vi "Time_Date_Data.vi"(8 "error in (no error)":errorcluster, 10 "SQL date time In":string, 11 "Serial Number":string) -> (0 "error out":errorcluster, 1 "WeekYearCode":string, 2 "UTC ISO 8601":string, 3 "time stamp":timestamp format="%<%H:%M:%S\n%d/%m/%Y>T", 4 "BTW WWYYSN":string, 5 "date time rec":T1, 6 "Sql datetime type 20":string, 7 "EMA time":string)   [LabVIEW 2013]
uses:
  <vilib>/Utility/miscctls.llb/LVDateTimeRec.ctl
  Main Support/Global 2.vi
panel:
  # "YYYYMMDDThhmmssZ"
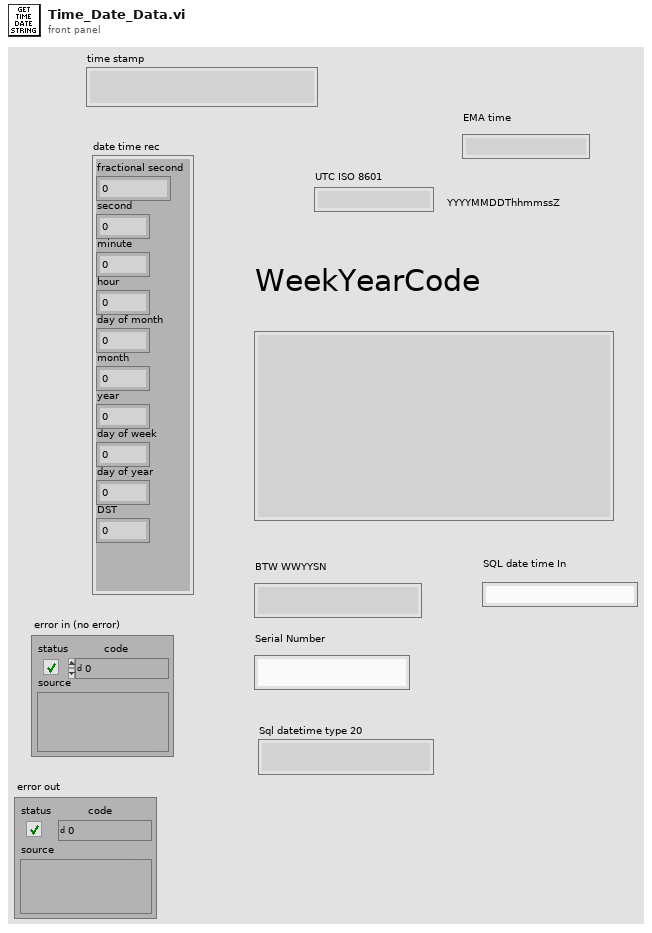
[diagram p1: front panel]
types:
  T1 = typedef "LVDateTimeRec.ctl" = cluster{"fractional second":dbl, "second":i32, "minute":i32, "hour":i32, "day of month":i32, "month":i32, "year":i32, "day of week":i32, "day of year":i32, "DST":i32}
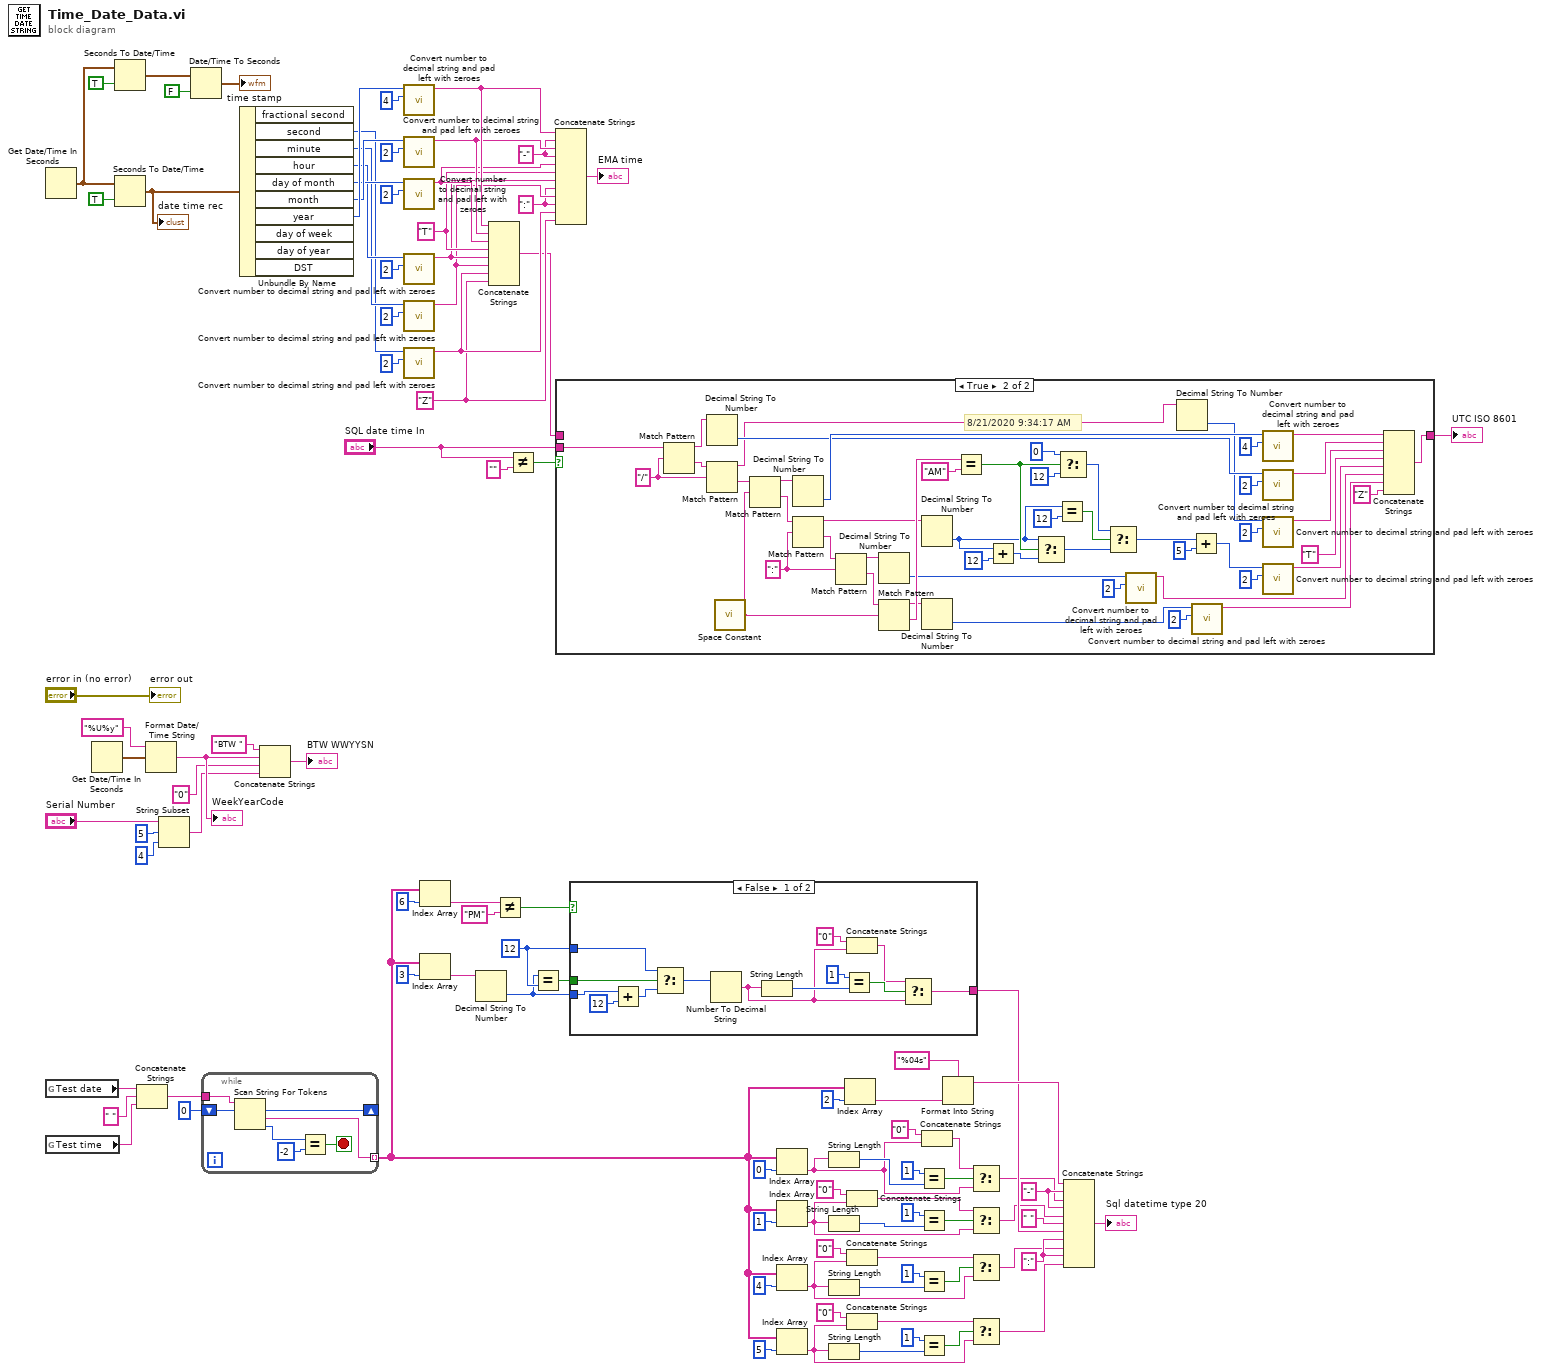
[diagram p0: block diagram]
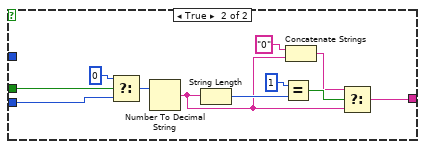
[diagram p3: hidden frame]
diagram:
  w9 = ":" ("string")
  w14 = "-" ("string")
  w50 = ":" ("string")
  w54 = "-" ("string")
  w56 = 12 ("y")
  w7 = "Z" ("string")
  w12 = "T" ("string")
  n1 = Get Date/Time In Seconds() -> (seconds since 1Jan1904=w96:timestamp)
  n2 = global read "Global 2.vi" "Test date"() -> (w20:string)
  n3 = global read "Global 2.vi" "Test time"() -> (w18:string)
  n4 = Get Date/Time In Seconds() -> (seconds since 1Jan1904=w94:timestamp)
  n5 = Seconds To Date/Time(time stamp (now)=w96, to UTC (F)=TRUE) -> (date time rec=w100:T1)
  n6 = Seconds To Date/Time(time stamp (now)=w96, to UTC (F)=TRUE) -> (date time rec=w95:T1)
  "date time rec" <- w95
  n7 = Concatenate Strings(w20, " " ("string"), w18) -> (w17:string)
  n8 = Format Date/Time String(time format string (%c)="%U%y", seconds (now)=w94) -> (date/time string=w91:string)  [unwired: 1 in]
  "WeekYearCode" <- w91
  n9 = String Subset(string="Serial Number", offset (0)=5, length (rest)=4 ("length (rest)")) -> (substring=w87:string)
  n10 = Date/Time To Seconds(1:FALSE ("to UTC (F)"), 2:w100) -> (0:→"time stamp":timestamp)
  n11 = while {
    tunnel: w17 -> [w109]
    shift-right: [w105] -> _
    shift-left: 0 -> [w106]
    tunnel: [w103] -> w61 mode=indexing
    stop <- w107 stop-if-true
    n12 = Scan String For Tokens(8:w106, 9:w109) -> (0:w104:i32, 1:w103:string, 2:w105:i32)  [unwired: 4 in, 1 out]
    n13 = Equal?(x=w104, y=-2) -> (x = y?=w107:bool)
  }
  n14 = Unbundle By Name(w95) -> ("second"=w74:i32, "minute"=w76:i32, "hour"=w78:i32, "day of month"=w80:i32, "month"=w82:i32, "year"=w84:i32)  [unwired: 4 out]
  n15 = Concatenate Strings("BTW " ("string"), w91, "0" ("string"), w87) -> (→"BTW WWYYSN":string)
  n16 = call "Convert number to decimal string and pad left with zeroes.vi"("Width"=u32 4, "number"=w84) -> ("result string"=w16:string)  [unwired: 9 in]
  n17 = call "Convert number to decimal string and pad left with zeroes.vi"("Width"=u32 2, "number"=w82) -> ("result string"=w15:string)  [unwired: 9 in]
  n18 = call "Convert number to decimal string and pad left with zeroes.vi"("Width"=u32 2, "number"=w80) -> ("result string"=w13:string)  [unwired: 9 in]
  n19 = call "Convert number to decimal string and pad left with zeroes.vi"("Width"=u32 2, "number"=w78) -> ("result string"=w11:string)  [unwired: 9 in]
  n20 = call "Convert number to decimal string and pad left with zeroes.vi"("Width"=i16 2 ("width (-)"), "number"=w76) -> ("result string"=w10:string)  [unwired: 9 in]
  n21 = call "Convert number to decimal string and pad left with zeroes.vi"("Width"=i16 2 ("width (-)"), "number"=w74) -> ("result string"=w8:string)  [unwired: 9 in]
  n22 = Index Array(array=w61, index=6) -> (element=w60:string)
  n23 = Index Array(array=w61, index=3) -> (element=w63:string)
  n24 = Decimal String To Number(string=w63) -> (number=w21:i32)  [unwired: 2 in, 1 out]
  n25 = Concatenate Strings(w16, w15, w13, w12, w11, w10, w8, w7) -> (w3:string)
  n26 = Not Equal?(x=w60, y="PM") -> (x != y?=w58:bool)
  n27 = Not Equal?(x="SQL date time In", y="") -> (x != y?=w4:bool)
  n28 = Equal?(x=w21, y=w56) -> (x = y?=w57:bool)
  n29 = Concatenate Strings(w16, w14, w15, w14, w13, w12, w11, w9, w10, w9, w8, w7) -> (→"EMA time":string)
  n30 = case shown="True" w4 {
    tunnel: w3 -> [w110 _]
    tunnel: [w110 w160] -> w2
    tunnel: "SQL date time In" -> [_ w158]
    frame False {
    }
    frame True {
      w152 = ":" ("regular expression")
      w156 = "/" ("regular expression")
      # "8/21/2020 9:34:17 AM"
      n31 = Match Pattern(string=w158, regular expression=w156) -> (before substring=w143:string, after substring=w157:string)  [unwired: 1 in, 2 out]
      n32 = Decimal String To Number(string=w143) -> (number=w145:i32)  [unwired: 2 in, 1 out]
      n33 = Match Pattern(string=w157, regular expression=w156) -> (before substring=w140:string, after substring=w155:string)  [unwired: 1 in, 2 out]
      n34 = call <vilib>:"Space Constant.vi"() -> ("String"=w150:string)
      n35 = Match Pattern(string=w155, regular expression=w150) -> (before substring=w147:string, after substring=w154:string)  [unwired: 1 in, 2 out]
      n36 = Decimal String To Number(string=w147) -> (number=w146:i32)  [unwired: 2 in, 1 out]
      n37 = Match Pattern(string=w154, regular expression=w152) -> (before substring=w138:string, after substring=w153:string)  [unwired: 1 in, 2 out]
      n38 = Match Pattern(string=w153, regular expression=w152) -> (before substring=w135:string, after substring=w151:string)  [unwired: 1 in, 2 out]
      n39 = Decimal String To Number(string=w135) -> (number=w137:i32)  [unwired: 2 in, 1 out]
      n40 = Match Pattern(string=w151, regular expression=w150) -> (before substring=w132:string, after substring=w149:string)  [unwired: 1 in, 2 out]
      n41 = Decimal String To Number(string=w138) -> (number=w116:i32)  [unwired: 2 in, 1 out]
      n42 = Decimal String To Number(string=w132) -> (number=w133:i32)  [unwired: 2 in, 1 out]
      n43 = Equal?(x=w149, y="AM") -> (x = y?=w117:bool)
      n44 = Add(x=w116, y=12) -> (x+y=w115:i32)
      n45 = Select(t=w116, s=w117, f=w115) -> (s? t:f=w114:i32)
      n46 = Equal?(x=w116, y=12) -> (x = y?=w122:bool)
      n47 = Select(t=u32 0 ("Width"), s=w117, f=12 ("y")) -> (s? t:f=w118:u32)
      n48 = Select(t=w118, s=w122, f=w114) -> (s? t:f=w111:u32)
      n49 = call "Convert number to decimal string and pad left with zeroes.vi"("Width"=u32 2, "number"=w137) -> ("result string"=w125:string)  [unwired: 9 in]
      n50 = Decimal String To Number(string=w140) -> (number=w141:i32)  [unwired: 2 in, 1 out]
      n51 = Add(x=w111, y=5) -> (x+y=w112:u32)
      n52 = call "Convert number to decimal string and pad left with zeroes.vi"("Width"=u32 2, "number"=w133) -> ("result string"=w124:string)  [unwired: 9 in]
      n53 = call "Convert number to decimal string and pad left with zeroes.vi"("Width"=u32 4, "number"=w146) -> ("result string"=w129:string)  [unwired: 9 in]
      n54 = call "Convert number to decimal string and pad left with zeroes.vi"("Width"=u32 2, "number"=w145) -> ("result string"=w128:string)  [unwired: 9 in]
      n55 = call "Convert number to decimal string and pad left with zeroes.vi"("Width"=u32 2, "number"=w141) -> ("result string"=w127:string)  [unwired: 9 in]
      n56 = call "Convert number to decimal string and pad left with zeroes.vi"("Width"=u32 2, "number"=w112) -> ("result string"=w126:string)  [unwired: 9 in]
      n57 = Concatenate Strings(w129, w128, w127, "T" ("string"), w126, w125, w124, "Z" ("string")) -> (w160:string)
    }
  }
  "UTC ISO 8601" <- w2
  n58 = case shown="False" w58 {
    tunnel: w57 -> [w173 w184]
    tunnel: w56 -> [w171 _]
    tunnel: [w162 w174] -> w52
    tunnel: w21 -> [w169 w182]
    frame False {
      n59 = Add(x=w169, y=12) -> (x+y=w172:i32)
      n60 = Select(t=w171, s=w173, f=w172) -> (s? t:f=w161:i32)
      n61 = Number To Decimal String(number=w161) -> (decimal integer string=w163:string)  [unwired: 1 in]
      n62 = String Length(string=w163) -> (length=w168:i32)
      n63 = Equal?(x=1, y=w168) -> (x = y?=w166:bool)
      n64 = Concatenate Strings("0" ("format string"), w163) -> (w164:string)
      n65 = Select(t=w164, s=w166, f=w163) -> (s? t:f=w162:string)
    }
    frame True {
      n66 = Select(t=i16 0 ("width (-)"), s=w184, f=w182) -> (s? t:f=w181:i32)
      n67 = Number To Decimal String(number=w181) -> (decimal integer string=w175:string)  [unwired: 1 in]
      n68 = String Length(string=w175) -> (length=w180:i32)
      n69 = Equal?(x=1, y=w180) -> (x = y?=w178:bool)
      n70 = Concatenate Strings("0" ("format string"), w175) -> (w176:string)
      n71 = Select(t=w176, s=w178, f=w175) -> (s? t:f=w174:string)
    }
  }
  n72 = Index Array(array=w61, index=0) -> (element=w44:string)
  n73 = Index Array(array=w61, index=1) -> (element=w37:string)
  n74 = Index Array(array=w61, index=4) -> (element=w30:string)
  n75 = Index Array(array=w61, index=5) -> (element=w23:string)
  n76 = String Length(string=w44) -> (length=w49:i32)
  n77 = String Length(string=w37) -> (length=w38:i32)
  n78 = String Length(string=w30) -> (length=w35:i32)
  n79 = String Length(string=w23) -> (length=w24:i32)
  n80 = Index Array(array=w61, index=2) -> (element=w67:string)
  n81 = Concatenate Strings("0" ("format string"), w37) -> (w42:string)
  n82 = Concatenate Strings("0" ("format string"), w30) -> (w31:string)
  n83 = Concatenate Strings("0" ("format string"), w23) -> (w28:string)
  n84 = Equal?(x=1, y=w49) -> (x = y?=w47:bool)
  n85 = Equal?(x=1, y=w38) -> (x = y?=w40:bool)
  n86 = Equal?(x=1, y=w35) -> (x = y?=w33:bool)
  n87 = Equal?(x=1, y=w24) -> (x = y?=w26:bool)
  n88 = Concatenate Strings("0" ("format string"), w44) -> (w45:string)
  n89 = Format Into String(format string="%04s", w67) -> (resulting string=w55:string)  [unwired: 2 in, 1 out]
  n90 = Select(t=w45, s=w47, f=w44) -> (s? t:f=w43:string)
  n91 = Select(t=w42, s=w40, f=w37) -> (s? t:f=w36:string)
  n92 = Select(t=w31, s=w33, f=w30) -> (s? t:f=w29:string)
  n93 = Select(t=w28, s=w26, f=w23) -> (s? t:f=w22:string)
  n94 = Concatenate Strings(w55, w54, w43, w54, w36, " " ("string"), w52, w50, w29, w50, w22) -> (→"Sql datetime type 20":string)
  "error out" <- "error in (no error)"
